vi "Memory.Pointer.Clear.Unsafe.vi"(8 "error in (no error)":errorcluster, 11 "pointer in":refnum<class "Memory.Pointer.lvclass">) -> (0 "error out":errorcluster, 3 "pointer out":refnum<class "Memory.Pointer.lvclass">)   [LabVIEW 2016, in "Memory Manager.lvlib" / "Memory.Pointer.lvclass"]
doc: "Sets the bytes specified by <b>pointer</b> to zero.\n\n<b>Note:</b> This VI is <b>unsafe</b>, meaning it does not performs null pointer and bounds checks to prevent invaid memory access. Invalid arguments provided to this method can crash or corrupt LabVIEW memory."
uses:
  Memory.Pointer.lvclass
  Memory.Pointer.lvclass/Memory.Pointer.ctl
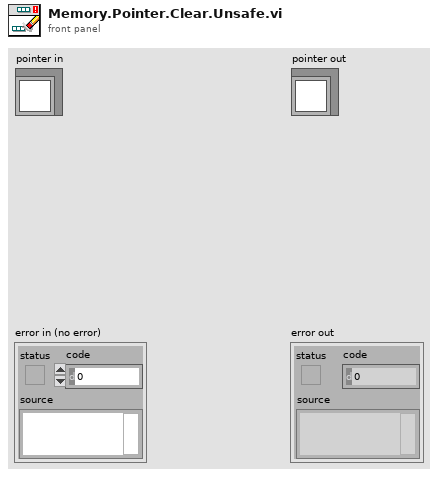
[diagram p1: front panel]
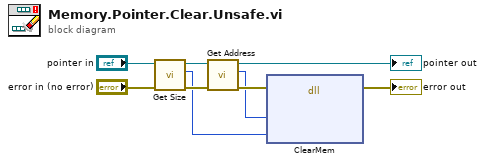
[diagram p0: block diagram]
diagram:
  n1 = call "Get Size.vi"("error in (no error)"="error in (no error)", "Pointer in"="pointer in") -> ("error out"=w6:errorcluster, "size"=w4:u64, "Pointer out"=w9:refnum<class "Memory.Pointer.lvclass">)  [unwired: 7 in]
  n2 = call "Get Address.vi"("error in (no error)"=w6, "Pointer in"=w9) -> ("error out"=w8:errorcluster, "address"=w3:u64, "Pointer out"=→"pointer out":refnum<class "Memory.Pointer.lvclass">)  [unwired: 7 in]
  n3 = dll-call lib="LabVIEW" fn="ClearMem"(error in=w8, "pointer"=w3, "size"=w4) -> (error out=→"error out":errorcluster)  [unwired: 5 in, 1 out]
